vi "reorderChannelsByBoard.vi"(11 "DAQmx \nPhysical Channel":tag="Dev2/ai0:31") -> (0 "Separated inputs\nas strings":string[](array[string]), 1 "number of boards used":i32, 2 "number \nchannels\nper board":i32[](array[numeric]))   [LabVIEW 2017]
doc: "Takes a list of channels and separates them into lists defined by their DAQ board. \nNecessary because labview can't read or write across channels from multiple boards with a single function call."
uses:
  <vilib>/Analysis/polynomials.llb/Unique Numbers and Multiplicity (DBL).vi
  <vilib>/regexp/Match Regular Expression.xnode
  <vilib>/Analysis/NI_AALPro.lvlib
panel:
  out "names out":string[](array[string])
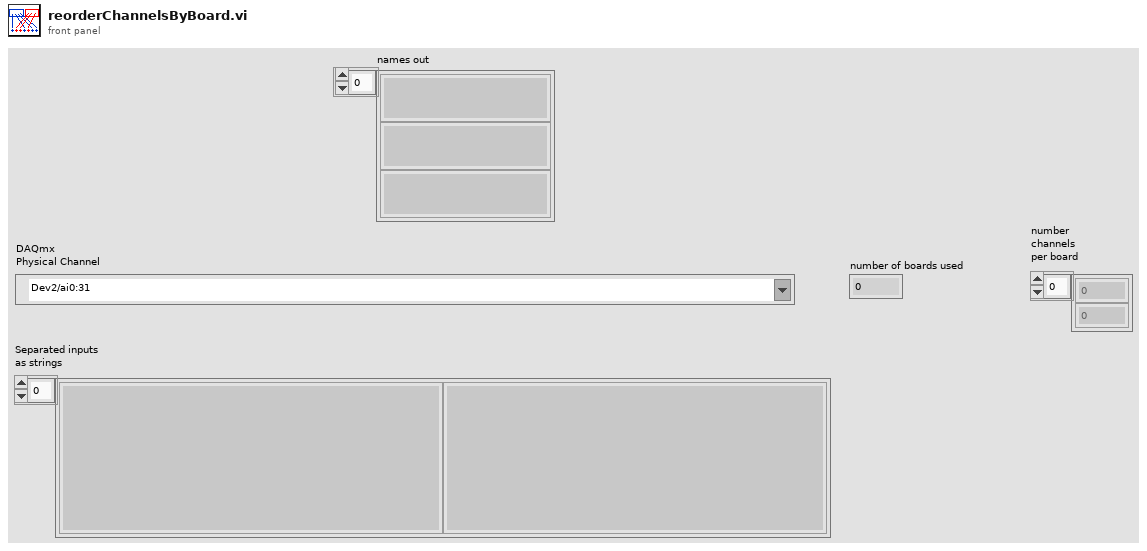
[diagram p1: front panel]
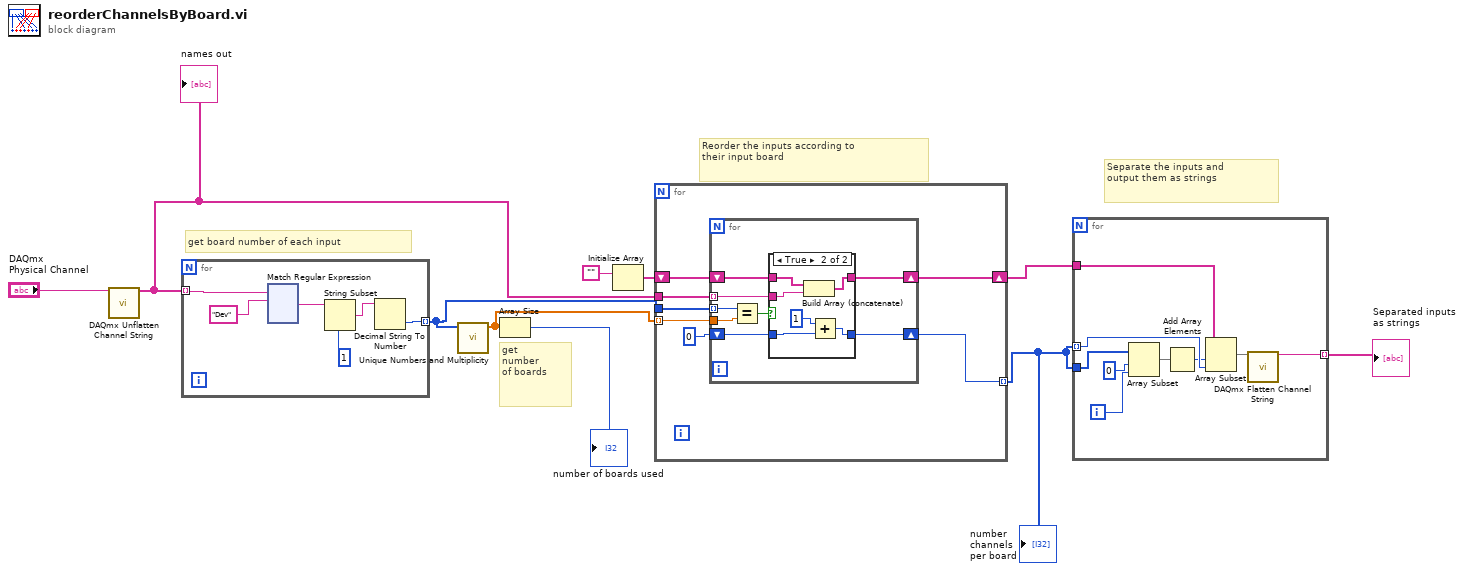
[diagram p0: block diagram]
diagram:
  # "Separate the inputs and \noutput them as strings"
  # "Reorder the inputs according to \ntheir input board"
  # "get \nnumber\nof boards"
  # "get board number of each input"
  n1 = call <vilib>:"DAQmx Unflatten Channel String.vi"("names in"="DAQmx \nPhysical Channel") -> ("names out"=w9:string[])  [unwired: 13 in, 1 out]
  "names out" <- w9
  n2 = for {
    tunnel: w9 -> [w14] mode=indexing
    tunnel: [w11] -> w8 mode=indexing
    n3 = xnode "Match Regular Expression"("input string"=w14, "regular expression"="Dev") -> ("after match"=w16:string)  [unwired: 4 in, 4 out]
    n4 = String Subset(string=w16, length (rest)=1 ("length (rest)")) -> (substring=w12:string)  [unwired: 1 in]
    n5 = Decimal String To Number(string=w12) -> (number=w11:i32)  [unwired: 2 in, 1 out]
  }
  n6 = call-poly <vilib>:"Unique Numbers and Multiplicity.vi"("Numbers"=w8) -> ("Unique Numbers"=w7:dbl[])  [unwired: 8 in, 2 out]
  n7 = Array Size(array=w7) -> (size(s)=→"number of boards used":i32)
  n8 = Initialize Array("") -> (w5:string[])  [unwired: 1 in]
  n9 = for {
    tunnel: w9 -> [w137]
    tunnel: w8 -> [w135]
    tunnel: w7 -> [w136] mode=indexing
    shift-right: [w133] -> w4
    shift-left: w5 -> [w134]
    tunnel: [w131] -> w2 mode=indexing
    n10 = for {
      tunnel: w137 -> [w144] mode=indexing
      shift-right: [w140] -> w133
      shift-left: w134 -> [w143]
      tunnel: w136 -> [w142]
      tunnel: w135 -> [w141] mode=indexing
      shift-right: [w138] -> w131
      shift-left: 0 -> [w139]
      n11 = Equal?(x=w141, y=w142) -> (x = y?=w145:bool)
      n12 = case shown="True" w145 {
        tunnel: w144 -> [_ w153]
        tunnel: [w147 w152] -> w140
        tunnel: w143 -> [w147 w151]
        tunnel: w139 -> [w146 w150]
        tunnel: [w146 w148] -> w138
        frame False {
        }
        frame True {
          n13 = Build Array (concatenate)(w151, w153) -> (w152:string[])
          n14 = Add(x=1, y=w150) -> (x+y=w148:i32)
        }
      }
    }
  }
  "number \nchannels\nper board" <- w2
  n15 = for {
    tunnel: w2 -> [w160]
    tunnel: w4 -> [w162]
    tunnel: w2 -> [w161] mode=indexing
    tunnel: [w154] -> w3 mode=indexing
    i -> [w156]
    n16 = Array Subset(array=w160, index=0, length=w156) -> (w158:i32[])
    n17 = Add Array Elements(numeric array=w158) -> (sum=w157:i32)
    n18 = Array Subset(array=w162, index=w157, length=w161) -> (w155:string[])
    n19 = call <vilib>:"DAQmx Flatten Channel String.vi"("names in"=w155) -> ("names out"=w154:string)  [unwired: 13 in, 1 out]
  }
  "Separated inputs\nas strings" <- w3
